vi "Read Stop Reason.vi"(8 "error in (no error)":errorcluster, 11 "Iterator Actor in":refnum<class "Iterator Actor.lvclass">) -> (0 "error out":errorcluster, 2 "Stop Reason":T1, 3 "Iterator Actor out":refnum<class "Iterator Actor.lvclass">)   [LabVIEW 2020, in "Iterator Actor.lvlib" / "Iterator Actor.lvclass"]
uses:
  Iterator Actor.lvclass
  Iterator Actor.lvclass/Iterator Actor.ctl
  Stop Reason.ctl
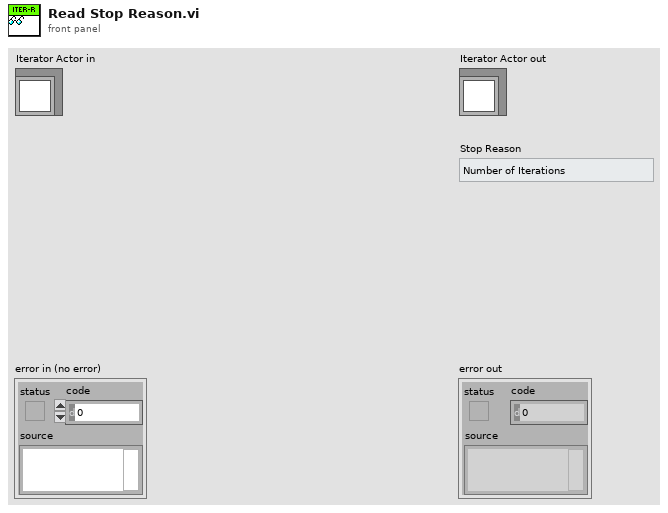
[diagram p1: front panel]
types:
  T1 = typedef "Iterator Actor.lvlib/Iterator Actor.lvclass/Stop Reason.ctl" = enum16{"Number of Iterations", "Time Elapsed", "Stopped Internally", "Stopped Externally"}
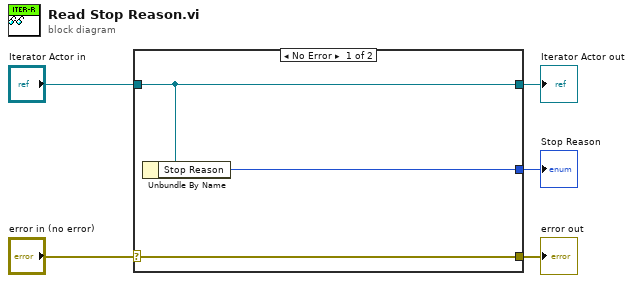
[diagram p0: block diagram]
diagram:
  n1 = case shown="No Error" "error in (no error)" {
    selector: "error in (no error)" -> [w8 w9]
    tunnel: [w8 w9] -> w4
    tunnel: [w7 w10] -> w2
    tunnel: "Iterator Actor in" -> [w7 w10]
    tunnel: [w6 _] -> w1
    frame No Error {
      n2 = Unbundle By Name(w7) -> ("Stop Reason"=w6:T1)
    }
    frame Error {
    }
  }
  "error out" <- w4
  "Iterator Actor out" <- w2
  "Stop Reason" <- w1
